vi "mupSetVarValue_Array.vi"(8 "error in (no error)":errorcluster, 10 "varValue":dbl[](array[numeric]), 11 "varPtr in":u64) -> (0 "error out":errorcluster, 3 "varPtr out":u64)   [LabVIEW 2015, in "mupLib.lvlib"]
uses:
  mupLib.lvlib
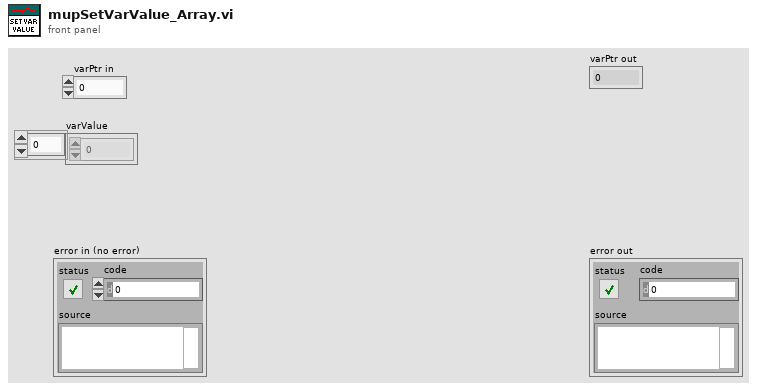
[diagram p1: front panel]
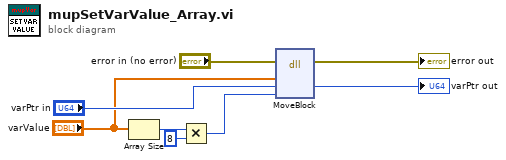
[diagram p0: block diagram]
diagram:
  n1 = Array Size(array="varValue") -> (size(s)=w8:i32)
  n2 = Multiply(x=w8, y=8) -> (x*y=w2:i32)
  n3 = dll-call lib="LabVIEW" fn="MoveBlock"(error in="error in (no error)", "ps"="varValue", "pd"="varPtr in", "size"=w2) -> (error out=→"error out":errorcluster, "pd"=→"varPtr out":u64)  [unwired: 5 in, 1 out]
